vi "Obtain Status.vi"(8 "error in (no error)":errorcluster, 11 "Home in":refnum<class "Home.lvclass">) -> (0 "error out":errorcluster, 1 "String":string, 2 "Page":T1(ring), 3 "Home out":refnum<class "Home.lvclass">)   [LabVIEW 2023, in "Home.lvclass"]
uses:
  Home.lvclass
  Home.lvclass/Home.ctl
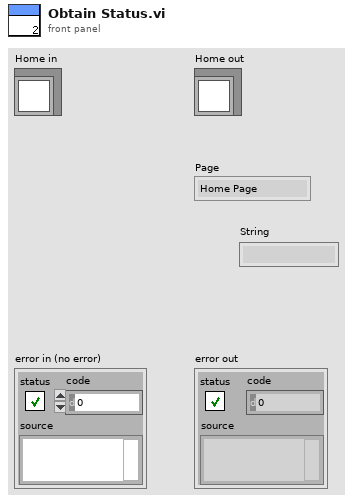
[diagram p1: front panel]
types:
  T1 = enum32{"Home Page", "Mode Page", "Configuration Page", "Input Page", "Result Page"}
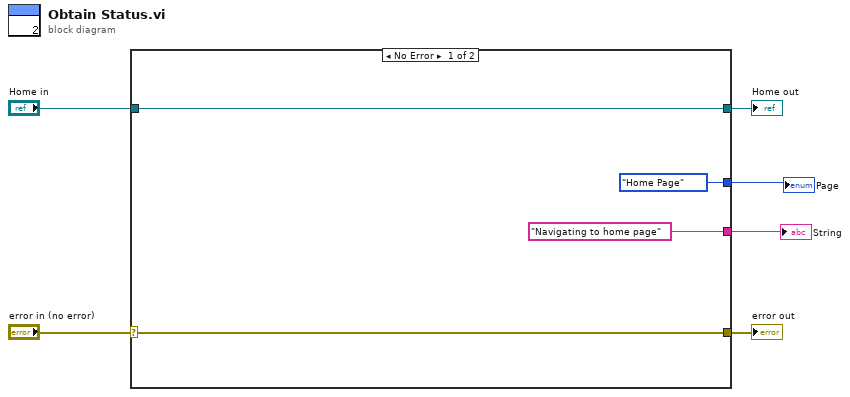
[diagram p0: block diagram]
diagram:
  n1 = case shown="No Error" "error in (no error)" {
    selector: "error in (no error)" -> [w9 w12]
    tunnel: [w9 w12] -> w5
    tunnel: [w10 w11] -> w3
    tunnel: "Home in" -> [w10 w11]
    tunnel: [T1."Home Page" ("Page") _] -> w2
    tunnel: ["Navigating to home page" _] -> w1
    frame No Error {
    }
    frame Error {
    }
  }
  "error out" <- w5
  "Home out" <- w3
  "Page" <- w2
  "String" <- w1
